vi "GPIB 332 Command.vi"(0 "GPIB (In)":cluster{"GPIB address":i16, "GPIB bus":i16}={"GPIB address"=15, "GPIB bus"=0}, 1 "Input command":string, 2 "error in":T1) -> (3 "GPIB (Out)":cluster{"GPIB address":i16, "GPIB bus":i16}={"GPIB address"=15, "GPIB bus"=0}, 4 "Bytes sent":i32, 5 "Return string":string, 6 "error out":T1)   [LabVIEW 2017]
doc: "Implements a GPIB command given the GPIB bus information and the input command string. The *OPC? query is sent after each command for handshaking purposes.\n\nMultiple serial polls are performed as required after sending the *OPC? command in order to determine when bit 4 (GPIB MESSAGE AVAILABLE) is set indicating the return data is available. Instruments must support the IEEE 488.2 spec for the serial poll byte for this VI to work correctly.\n\nThe *OPC? timeout setting (internal to VI) limits the amount of time the VI will wait for bit 4 to be set by the instrument."
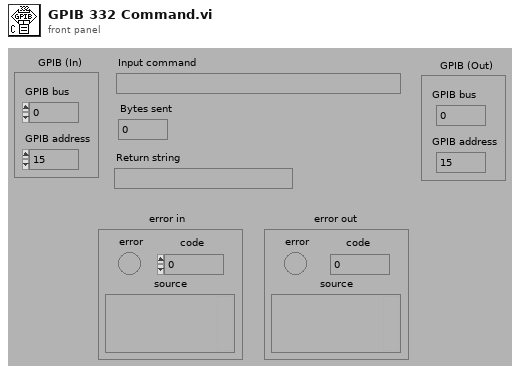
[diagram p1: front panel]
types:
  T1 = cluster{"error":bool, "code":i32, "source":string}
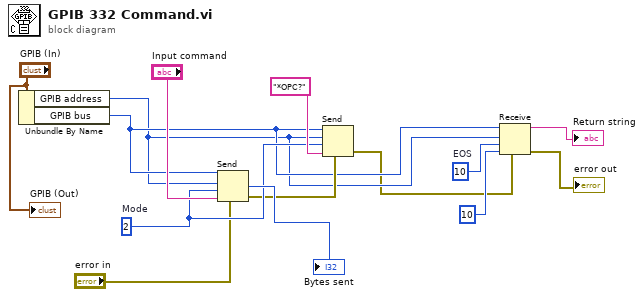
[diagram p0: block diagram]
diagram:
  w2 = u8 10  # EOS
  w9 = u8 2  # Mode
  n1 = Unbundle By Name("GPIB (In)") -> ("GPIB address"=w3:i16, "GPIB bus"=w4:i16)
  n2 = Send(0:w4, 2:w3, 3:w9, 4:"error in", 5:"Input command") -> (7:→"Bytes sent":i32, 8:w7:errorcluster)  [unwired: 1 out]
  n3 = Send(0:w4, 2:w3, 3:w9, 4:w7, 5:"*OPC?") -> (8:w1:errorcluster)  [unwired: 2 out]
  n4 = Receive(4:w1, 6:10, 7:w2, 8:w3, 9:w4) -> (0:→"error out":errorcluster, 3:→"Return string":string)  [unwired: 2 out]
  "GPIB (Out)" <- "GPIB (In)"
